vi "STRLEN.vi"(0 "refnum in":refnum<vi>, 1 "Key":string, 11 "error in":errorcluster) -> (4 "refnum out":refnum<vi>, 6 "Data":T1, 15 "error out":errorcluster)   [LabVIEW 2020]
uses:
  SubVIs/Controls/redis-data.ctl
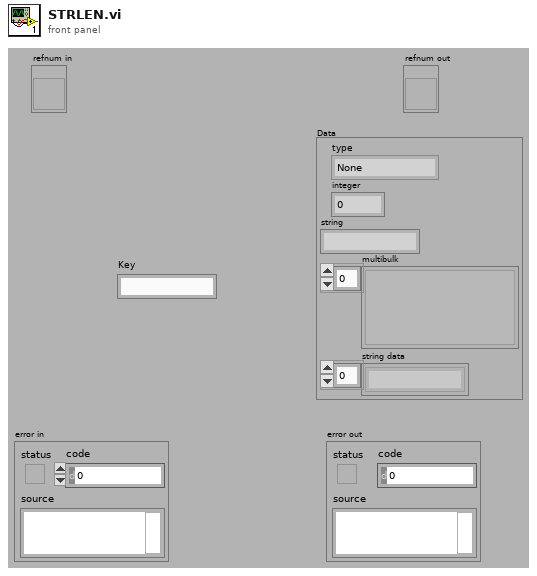
[diagram p1: front panel]
types:
  T1 = typedef "redis-data.ctl" = cluster{"type":enum16{"None", "Error", "Status", "Nil", "Integer", "String", "Multibulk"}, "integer":i64, "string":string, "multibulk":variant[], "string data":string[]}
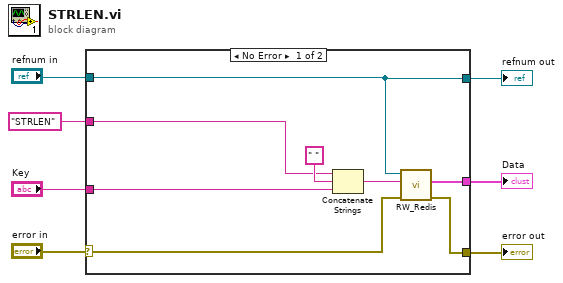
[diagram p0: block diagram]
diagram:
  n1 = case shown="No Error" "error in" {
    selector: "error in" -> [w12 w17]
    tunnel: "Key" -> [w9 _]
    tunnel: "STRLEN" -> [w14 _]
    tunnel: "refnum in" -> [w8 w16]
    tunnel: [w11 w17] -> w5
    tunnel: [w10 _] -> w1
    tunnel: [w8 w16] -> w2
    frame No Error {
      n2 = Concatenate Strings(w14, " ", w9) -> (w13:string)
      n3 = call "RW_Redis.vi"("error in"=w12, "command"=w13, "refnum"=w8) -> ("error out"=w11:errorcluster, "Data"=w10:T1)  [unwired: 7 in]
    }
    frame Error {
    }
  }
  "error out" <- w5
  "refnum out" <- w2
  "Data" <- w1
